vi "Get Monitor DPI.vi"(8 "error in (no error)":errorcluster, 11 "hMon":u32) -> (0 "error out":errorcluster, 2 "DPI":i32, 3 "hMon out":u32)   [LabVIEW 2020, in "MacroAssert.lvlib" / "Win Util.lvlib"]
doc: "Outputs the display scale, in percent, of the monitor identified by <B>hMon</B>."
uses:
  Win Util.lvlib
  SHCore.dll
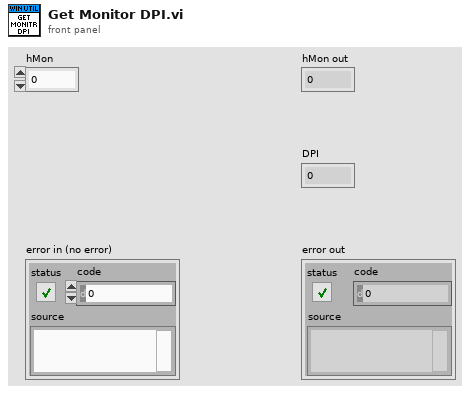
[diagram p1: front panel]
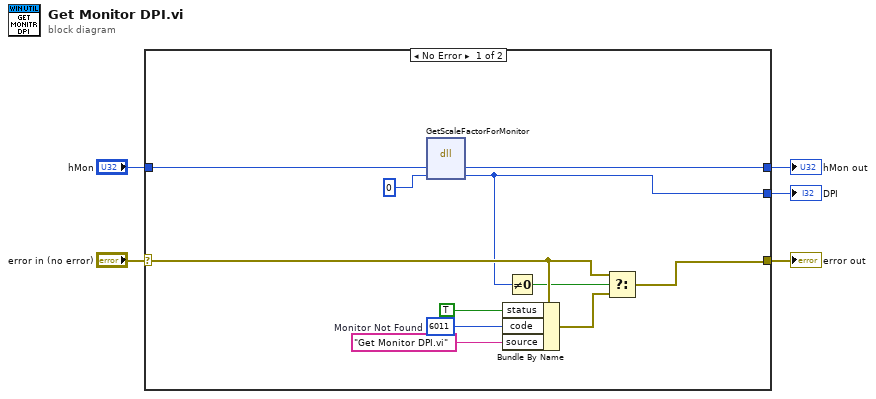
[diagram p0: block diagram]
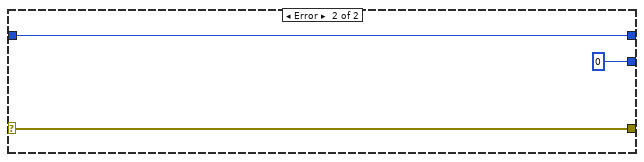
[diagram p2: hidden frame]
diagram:
  n1 = case shown="No Error" "error in (no error)" {
    selector: "error in (no error)" -> [w16 w19]
    tunnel: [w15 w19] -> w4
    tunnel: [w14 0] -> w3
    tunnel: "hMon" -> [w6 w17]
    tunnel: [w7 w17] -> w1
    frame No Error {
      w10 = 6011  # Monitor Not Found
      n2 = dll-call lib="SHCore.dll" fn="GetScaleFactorForMonitor"("hMon"=w6, "pScale"=0) -> ("hMon"=w7:u32, "pScale"=w14:i32)  [unwired: 3 in, 3 out]
      n3 = Bundle By Name(cluster=w16, "status"=TRUE ("show call chain? (False)"), "code"=w10, "source"="Get Monitor DPI.vi") -> (w8:errorcluster)
      n4 = Not Equal To 0?(x=w14) -> (x != 0?=w12:bool)
      n5 = Select(t=w16, s=w12, f=w8) -> (s? t:f=w15:errorcluster)
    }
    frame Error {
    }
  }
  "error out" <- w4
  "DPI" <- w3
  "hMon out" <- w1
